vi "Init.vi"(10 "Player ID":i32, 11 "BTeam in":refnum<class "BTeam.lvclass">) -> (1 "X Loc":i32, 2 "Y Loc":i32, 3 "BTeam out":refnum<class "BTeam.lvclass">)   [LabVIEW 2015, in "BTeam.lvclass"]
uses:
  BTeam.lvclass
  Team Cluster.ctl
  Mode Enum.ctl
  BTeam.lvclass/BTeam.ctl
  TeamEffort/TeamEffort.lvclass
  Square/Square.lvclass
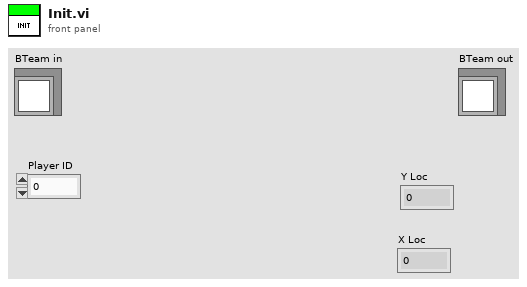
[diagram p1: front panel]
types:
  T1 = typedef "BTeam.lvclass/Mode Enum.ctl" = enum16{"<Unknown>", "1", "2", "4", "8", "16", "Check", "Spawn"}
  T2 = typedef "BTeam.lvclass/Team Cluster.ctl" = cluster{"Mode":T1, "Y":i32, "X":i32, "Count":i32, "Dir":i32}
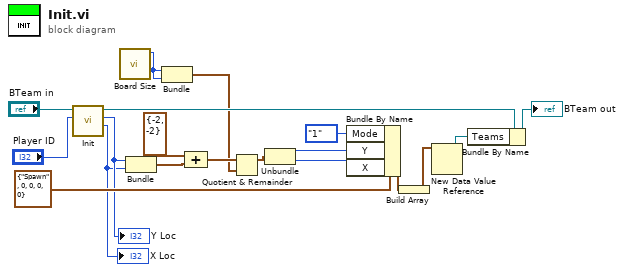
[diagram p0: block diagram]
diagram:
  n1 = call-parent "Init.vi"("Player ID"="Player ID", "TeamEffort in"="BTeam in") -> ("X Loc"=w10:i32, "Y Loc"=w11:i32, "TeamEffort out"=w15:refnum<class "BTeam.lvclass">)  [unwired: 7 in]
  "X Loc" <- w10
  "Y Loc" <- w11
  n2 = call "Board Size.vi"() -> ("Board Size"=w7:i32)  [unwired: 11 in]
  n3 = Bundle("Y Loc"=w11, "X Loc"=w10) -> (w9:cluster{"Y Loc":i32, "X Loc":i32})  [unwired: 1 in]
  n4 = Bundle("Board Size"=w7, "Board Size"=w7) -> (w5:cluster{"Board Size":i32, "Board Size":i32})  [unwired: 1 in]
  n5 = Compound Arithmetic op=ADD(cluster{"Y Loc":i32, "X Loc":i32} {"Y Loc"=-2, "X Loc"=-2} ("x"), w9) -> (w6:cluster{"Y Loc":i32, "X Loc":i32})
  n6 = Quotient & Remainder(x=w6, y=w5) -> (x-y*floor(x/y)=w4:cluster{i32, i32})  [unwired: 1 out]
  n7 = Unbundle(w4) -> (w3:i32, w2:i32)
  n8 = Bundle By Name(cluster=T2 {"Mode"=enum."Spawn", "Y"=0, "X"=0, "Count"=0, "Dir"=0} ("Team Cluster"), "Mode"=Mode_Enum."1", "Y"=w3, "X"=w2) -> (w12:T2)
  n9 = Build Array(w12) -> (w16:T2[])
  n10 = New Data Value Reference(data value=w16) -> (data value reference=w14:refnum<data-value>)  [unwired: 1 in, 1 out]
  n11 = Bundle By Name(cluster=w15, "Teams"=w14) -> (→"BTeam out":refnum<class "BTeam.lvclass">)
